vi "HWhist-TimeSeriesStrictTiming.vi"() -> ()   [LabVIEW 2017]
doc: "This example demonstrates how to use the Becker&Hickl LabVIEW wrapper VIs to acquire decay curves in continuous flow mode using the sequencer and swapping banks.\nMultiple modules are covered in a parallelized for loop.\nEach bank's decay curves are saved to a SDT-file on disc.\nThe SPC parameters can be adjusted for every new run. The rates and status flags are continuously updated. This VI is based on the C-example part 1 in use_spcm.c\n\ninfo@becker-hickl.com"
uses:
  Example_Controls/UserInput-PerModules.ctl
  Example_Controls/UserInput-AllModules.ctl
  SPC_Wrappers/SPC_Controls/ADCResolution.ctl
  SPC_Wrappers/SPC_Controls/StateCluster.ctl
  Example_Controls/CFM_States.ctl
  SPC_Wrappers/SPC_Controls/dither_range.ctl
  SPC_Wrappers/SPC_Controls/SPCdata.ctl
  SPC_Wrappers/SPC_Controls/macro_time_clk.ctl
  SPC_Wrappers/SPC_Controls/par_id.ctl
panel:
  out "Measurement Time":dbl(knob) scale=0.0..153.59999084472656
  out "CurrentBank":sgl
  out "SavingTime[s]":dbl
  out "saving":bool[](array[boolean])
  out "collecting":bool[](array[boolean])
  out "Busy":bool
  out "Sync Status":bool=TRUE
  in  "Tab Control":T1(tab)
  in  "User Input AllModules":T2={"tac_range"=50.033573, "tac_gain"=1, "tac_offset"=0.0, "tac_limit_high"=100.0, "tac_limit_low"=0.0, "collect_time"=0.1} {"tac_limit_high" min=0 max=100 step=0.1; "collect_time" min=1e-07 max=100000 step=0.001; "tac_offset" min=0 max=100 step=0.1; "tac_gain" min=1 max=15 step=1; "tac_range" format="%^#_6g"}
  in  "No of Routing Channels":i16(ring)=1 items=["1"=1, "2"=2, "3"=3, "4"=4, "5"=5, "6"=6, "7"=7, "8"=8, "9"=9, "10"=10, "11"=11, "12"=12, "13"=13, "14"=14, "15"=15, "16"=16]
  in  "ADC Resolution":T3=12 items=["1"=0, "4"=2, "16"=4, "64"=6, "256"=8, "1024"=10, "4096"=12]
  in  "User Input PerModule":T4[](array[typedef])=[{"sync_threshold"=-50.0, "sync_zc_level"=-5.2999988, "sync_freq_div"=1, "cfd_limit_low"=-50.0, "cfd_zc_level"=5.3000016}, {"sync_threshold"=-50.0, "sync_zc_level"=-5.2999988, "sync_freq_div"=1, "cfd_limit_low"=-50.0, "cfd_zc_level"=5.3}] {"sync_freq_div" items=["1"=1, "2"=2, "4"=4]; "cfd_zc_level" min=-96 max=96 step=0.1 format="%#_3g"; "cfd_limit_low" min=-500 max=0 step=0.1 format="%#_3g"; "sync_zc_level" min=-96 max=96 step=0.1 format="%#_3g"; "sync_threshold" min=-500 max=-20 step=0.1 format="%#_3g"}
  in  "Use First Entry\nFor All Modules":bool=TRUE
  out "Sync Array":T5(array[cluster])=[{"Sync Rate"=49999104.0, TRUE, "CFD Rate"=548976.0, "TAC Rate"=517664.0, "ADC Rate"=0.0}, {"Sync Rate"=49999360.0, TRUE, "CFD Rate"=544768.0, "TAC Rate"=514432.0, "ADC Rate"=0.0}]
  out "State Array":T6[](array[typedef])
  in  "ActiveModules":i32[](listbox)
  out "Data":u16[][](graph) caption="FirstCurve only"
  out "IntensityGraph":cluster{"Intensity Graph":u16[][]}[](array[cluster])
  in  "Saving Path":path=path "c:/temp"
  in  "Stop Application":bool
  out "Cycle Process":dbl(slide)=10.0 scale=0.0..100.0
  in  "CountCycles":bool=TRUE
  out "Current Cycle":i32=1
  in  "Number of\nCycles":i32=3
  in  "Stop Measurement":bool
  in  "Start Measurement":bool
  out "Started at":timestamp=timestamp(3689245583.9141345 s since 1904-01-01)
  out "Estimated Duration\nper Bank [min]":sgl=0.85333335
  out "Estimated Duration\nper Bank [s]":sgl=51.2
  out "Active Module No":i16[](array[numeric])=[0, 1]
  # "This example demonstrates how to use the Becker&Hickl LabVIEW wrapper VIs to acquire decay curves in continuous flow mode using the sequencer and swapping banks.\nMultiple modules are covered in a parallelized for loop.\nEach bank's decay curves are saved to a SDT-file on disc.\nThe SPC parameters can be adjusted for every new run. The rates and status flags are continuously updated.              This VI is based on the C-example part 1 in use_spcm.c."
  # "TAC / Time Range"
  # "range"
  # "gain"
  # "offset"
  # "limit high"
  # "limit low"
  # "Collection Time"
  # "CFD"
  # "(start)"
  # "SYNC"
  # "(stop)"
  # "threshold(LL)"
  # "zero cross(ZC)"
  # "See Tip-Strip for details"
  # "(c) 2022 Becker & Hickl GmbH\n     ALL RIGHTS RESERVED."
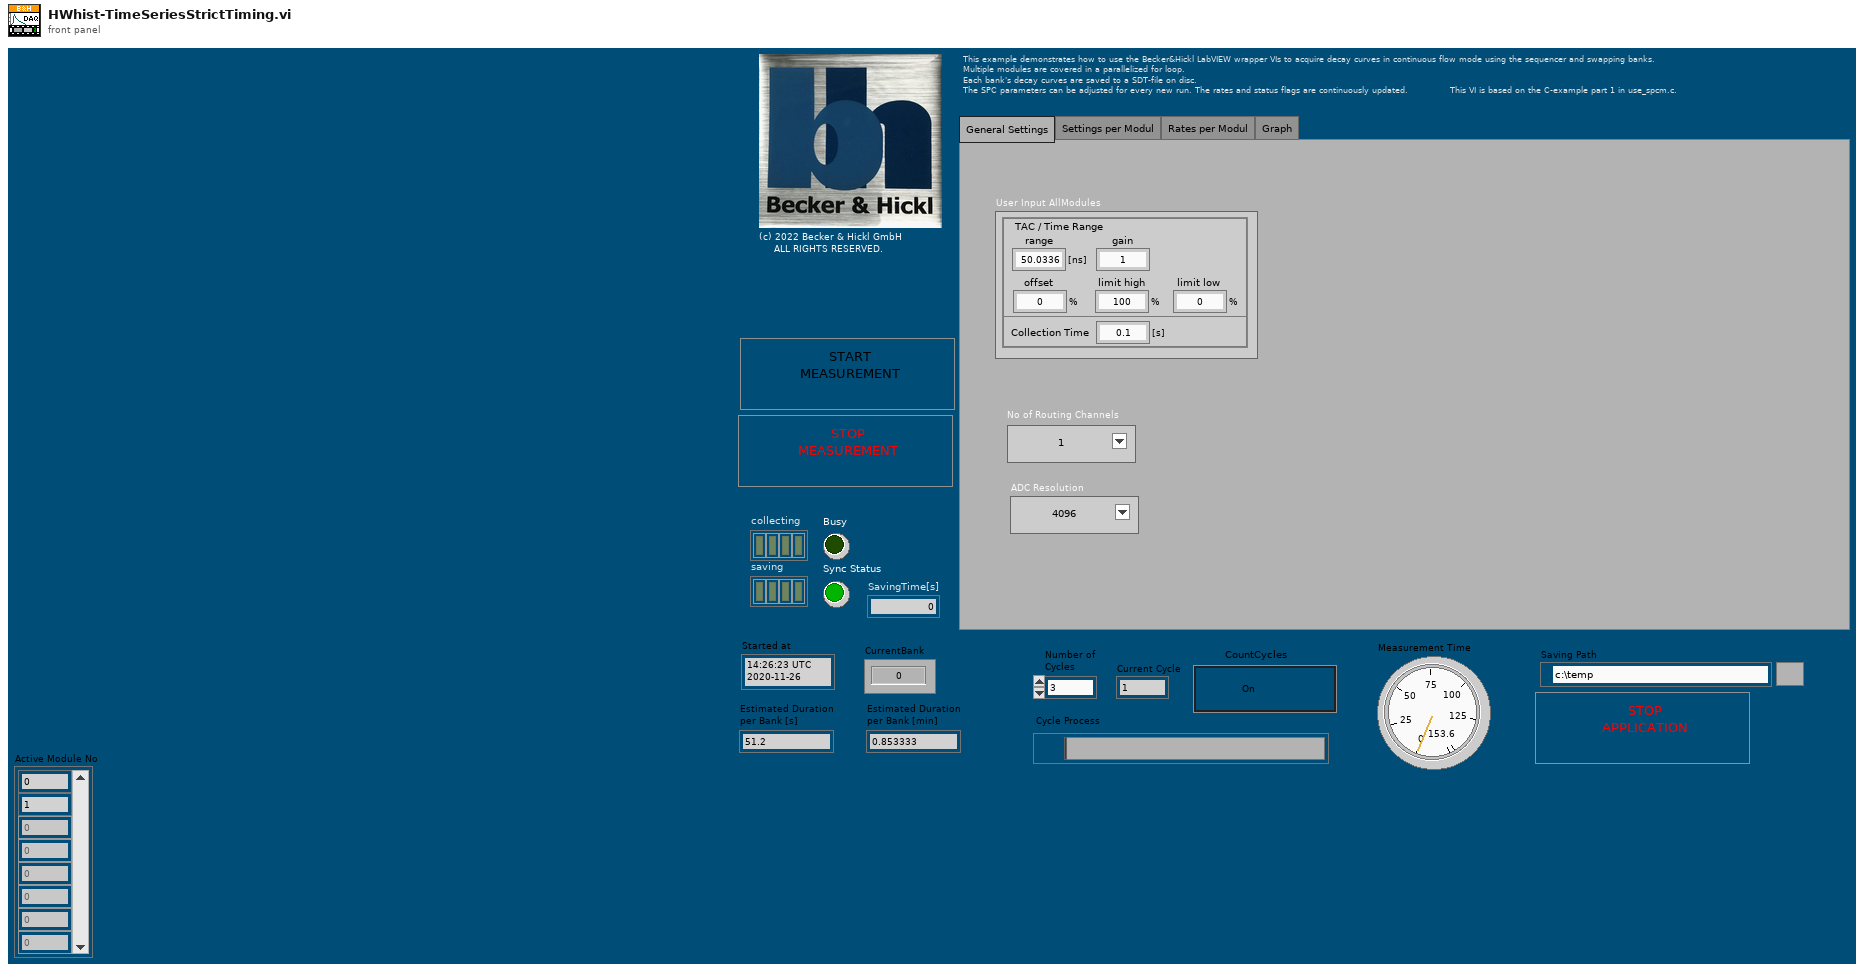
[diagram p1: front panel]
types:
  T1 = enum32{"General Settings", "Settings per Modul", "Rates per Modul", "Graph"}
  T2 = typedef "UserInput-AllModules.ctl" = cluster{"tac_range":sgl, "tac_gain":i16, "tac_offset":sgl, "tac_limit_high":sgl, "tac_limit_low":sgl, "collect_time":sgl}
  T3 = typedef "ADCResolution.ctl" = i16
  T4 = typedef "UserInput-PerModules.ctl" = cluster{"sync_threshold":sgl, "sync_zc_level":sgl, "sync_freq_div":i16, "cfd_limit_low":sgl, "cfd_zc_level":sgl}
  T5 = cluster{"Sync Rate":sgl, bool, "CFD Rate":sgl, "TAC Rate":sgl, "ADC Rate":sgl}[]
  T6 = typedef "StateCluster.ctl" = cluster{"OVERFL":bool, "OVERFLOW":bool, "TIME_OVER":bool, "COLTIM_OVER":bool, "CMD_STOP":bool, "ARMED":bool, "REPTIM_OVER":bool, "COLTIM_2OVER":bool, "REPTIM_2OVER":bool, "FOVFL":bool, "FEMPTY":bool, "FBRDY":bool, "SCRDY":bool, "MEASURE":bool, "WAIT_TRG":bool, "HFILL_NRDY":bool, "SEQ_STOP":bool, "SEQ_GAP150":bool, "WAIT_FR":bool}
  T7 = typedef "macro_time_clk.ctl" = enum16{"25ns", "Sync", "1/2 Sync", "1/4 Sync", "1/8 Sync"}
  T8 = typedef "SPCdata.ctl" = cluster{"base_adr":u16, "init":i16, "cfd_limit_low":sgl, "cfd_limit_high":sgl, "cfd_zc_level":sgl, "cfd_holdoff":sgl, "sync_zc_level":sgl, "sync_holdoff":sgl, "sync_threshold":sgl, "tac_range":sgl, "sync_freq_div":i16, "tac_gain":i16, "tac_offset":sgl, "tac_limit_low":sgl, "tac_limit_high":sgl, "adc_resolution":i16, "ext_latch_delay":i16, "collect_time":sgl, "display_time":sgl, "repeat_time":sgl, "stop_on_time":i16, "stop_on_ovfl":i16, "dither_range":i16, "count_incr":i16, "mem_bank":i16, "dead_time_comp":i16, "scan_control":u16, "routing_mode":u16, "tac_enable_hold":sgl, "pci_card_no":i16, "mode":u16, "scan_size_x":u32, "scan_size_y":u32, "scan_rout_x":u32, "scan_rout_y":u32, "scan_flyback":u32, "scan_borders":u32, "scan_polarity":u16, "pixel_clock":u16, "line_compression":u16, "trigger":u16, "pixel_time":sgl, "ext_pixclk_div":u32, "rate_count_time":sgl, "macro_time_clk":i16, "add_select":i16, "test_eep":i16, "adc_zoom":i16, "img_size_x":u32, "img_size_y":u32, "img_rout_x":u32, "img_rout_y":u32, "xy_gain":i16, "master_clock":i16, "adc_sample_delay":i16, "detector_type":i16, "chan_enable":u32, "chan_slope":u32, "chan_spec_no":u32, "tdc_control":u32, "tdc_offset1":sgl, "tdc_offset2":sgl, "tdc_offset3":sgl, "tdc_offset4":sgl, "tdc_offset5":sgl, "tdc_offset6":sgl, "cfd_th5_tdc":sgl, "cfd_th6_tdc":sgl, "cfd_zc5_tdc":sgl, "cfd_zc6_tdc":sgl, "future_reserve1":u64, "future_reserve2":u64, "future_reserve3":u64, "future_reserve4":u64}
  T9 = typedef "dither_range.ctl" = i16
  T10 = typedef "CFM_States.ctl" = enum16{"Init", "IDLE", "PrepareMeasurement", "StartMeasurement"}
  T11 = typedef "SPCModInfo.ctl" = cluster{"Module Type":T12, "Bus Number":i16, "Slot Number":i16, "in Use":i16, "Init Status":i16, "Base I/O Addr":u16}
  T12 = typedef "ModuleType.ctl" = i16
  T13 = typedef "ConfigMem.ctl" = cluster{"Max Block No":i32, "Blocks Per Frame":i32, "Frames Per Page":i32, "Maxpage":i32, "Block Length":i32}
  T14 = typedef "par_id.ctl" = i16
  T15 = typedef "SPC_RatesCluster.ctl" = cluster{"Sync":sgl, "CFD":sgl, "TAC":sgl, "ADC":sgl}
  T16 = cluster{"Sync":sgl, bool, "CFD":sgl, "TAC":sgl, "ADC":sgl}
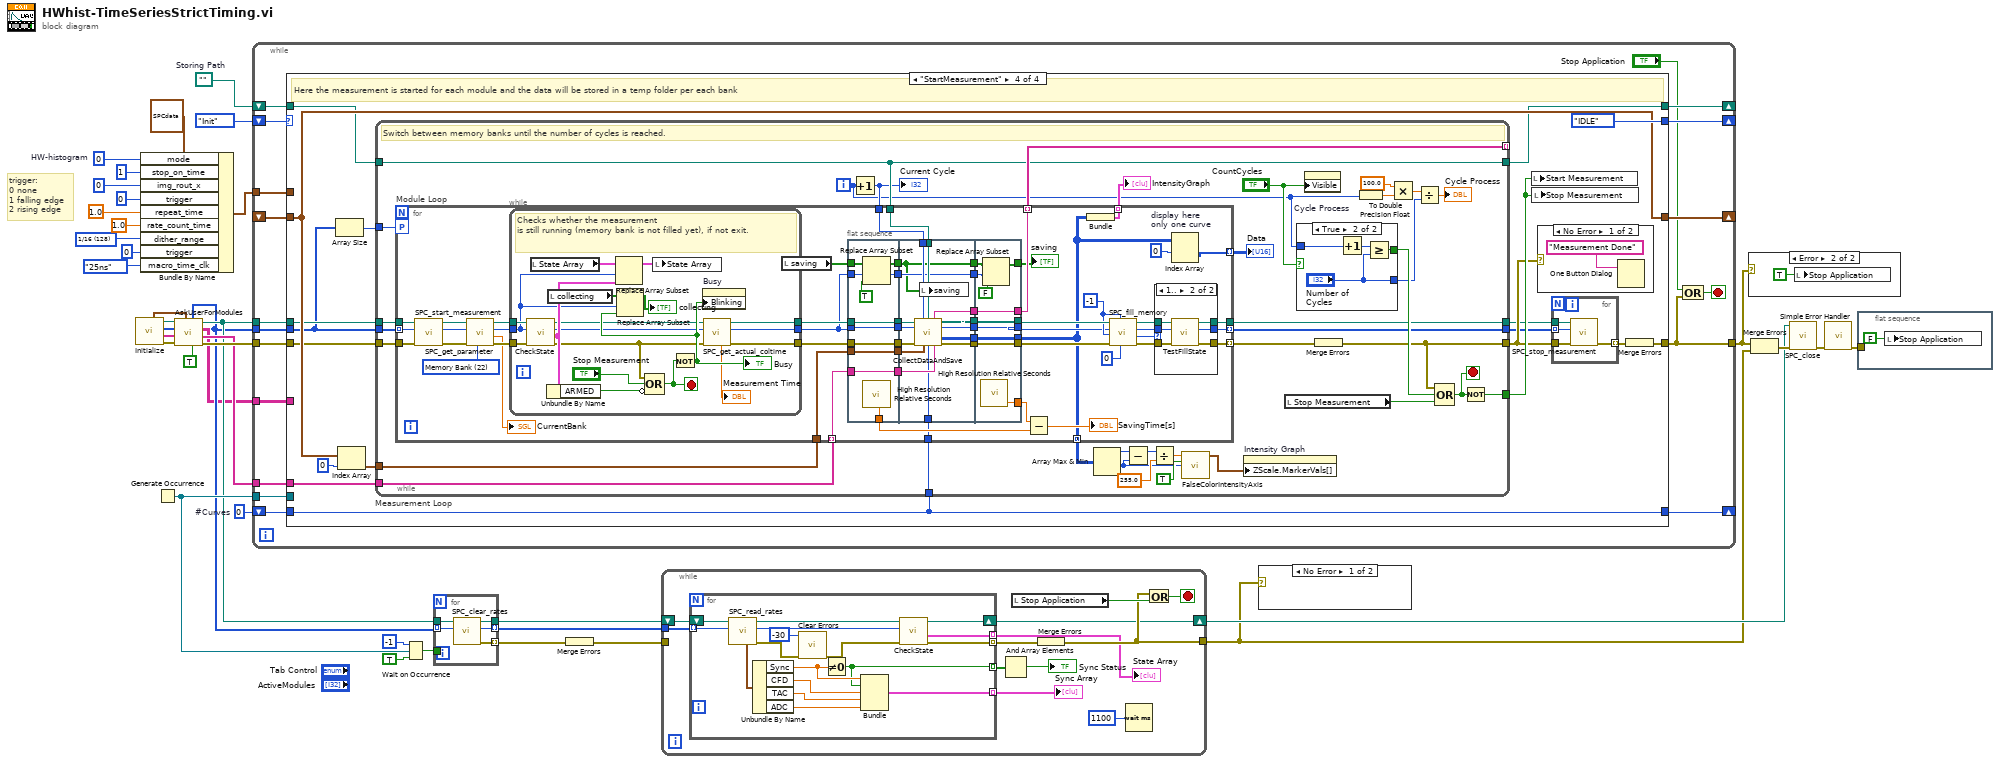
[diagram p0: block diagram]
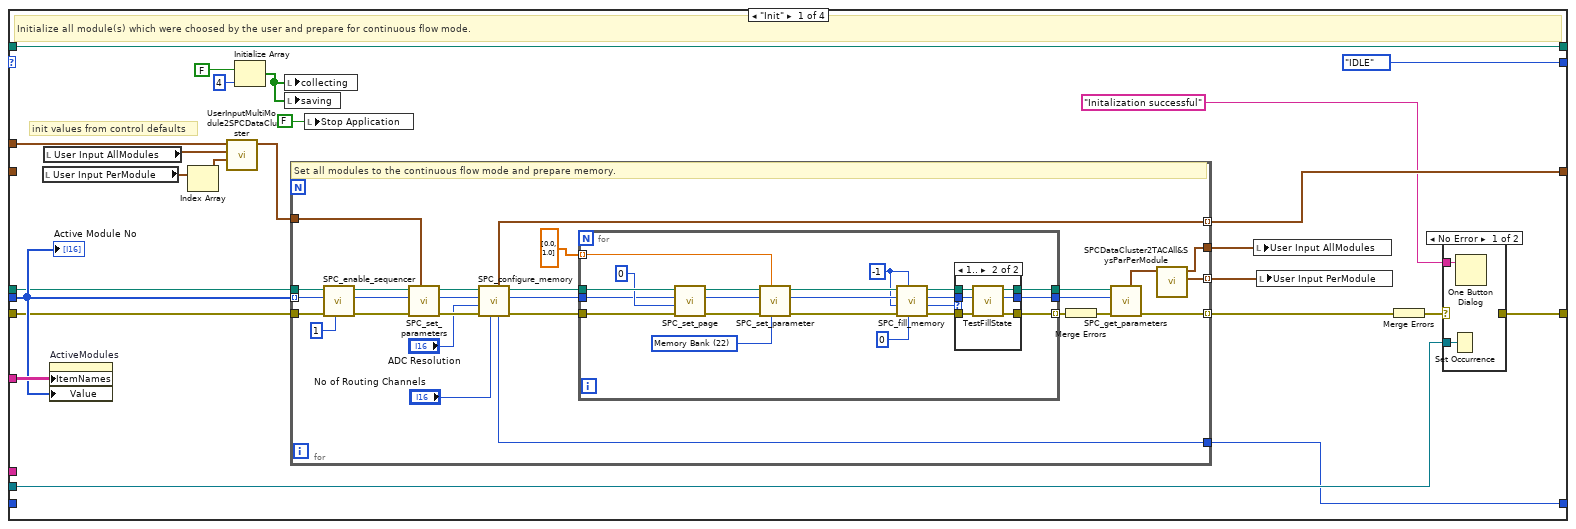
[diagram p2: hidden frame]
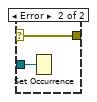
[diagram p3: hidden frame]
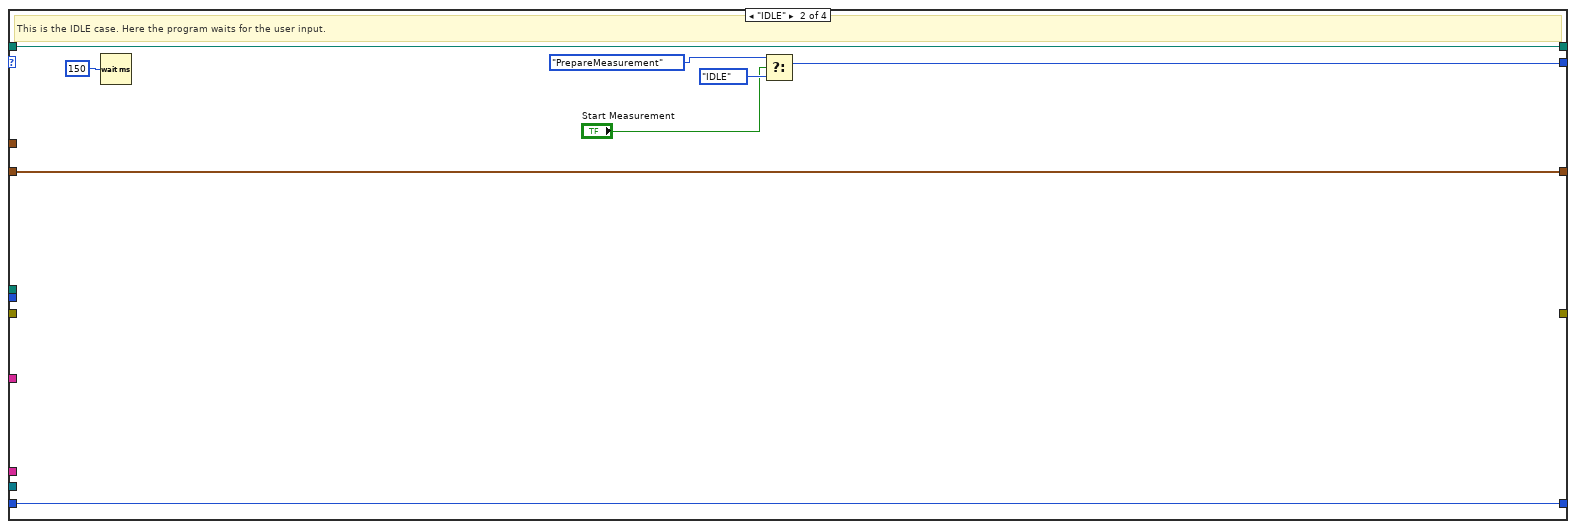
[diagram p5: hidden frame]
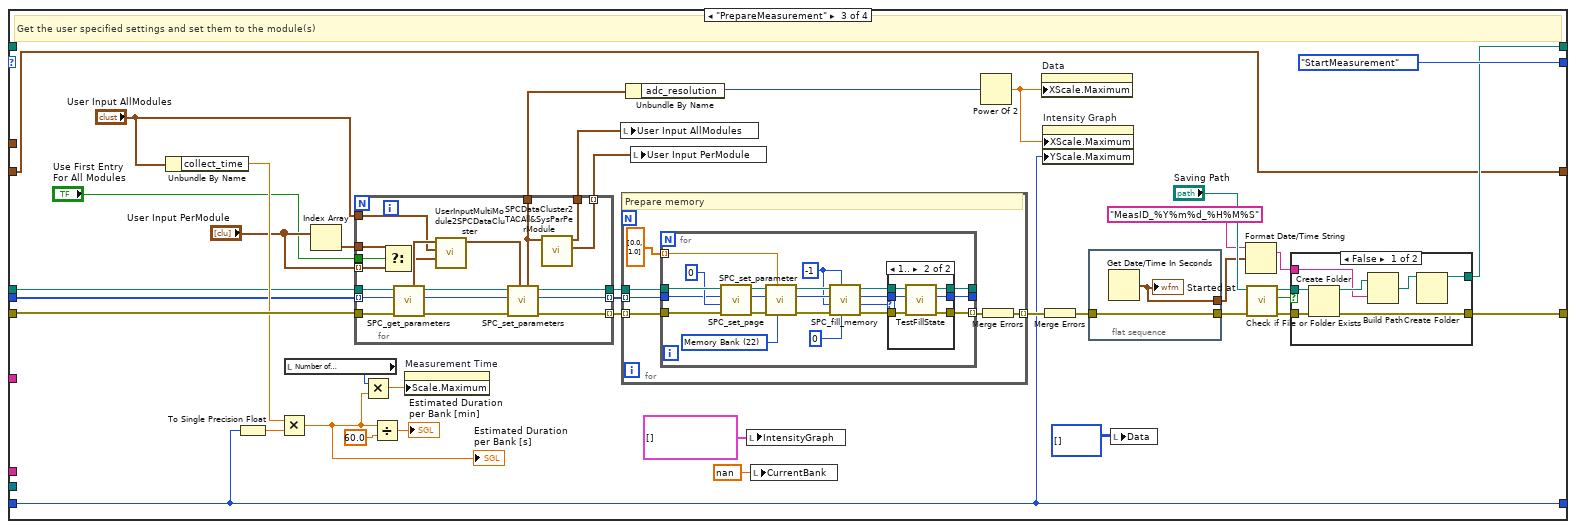
[diagram p6: hidden frame]
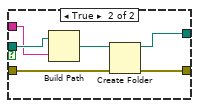
[diagram p8: hidden frame]
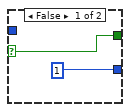
[diagram p11: hidden frame]
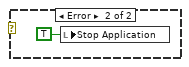
[diagram p12: hidden frame]
diagram:
  w4 = T9 128 items=["0"=0, "1/64"=32, "1/32"=64, "1/16"=128, "1/8"=256] ("DithRange")
  w12 = u16 0  # HW-histogram
  w17 = 0  # #Curves
  w35 = path ""  # Storing Path
  # "trigger:\n0 none\n1 falling edge\n2 rising edge"
  n1 = call "Initialize.vi"() -> ("ErrorOut"=w29:errorcluster, "SerialNumbersArray"=w24:string[], "ModuleNoArray"=w25:i16[], "DLL Path"=w33:path, "SPCModulesArray"=w23:T11[])  [unwired: 7 in]
  n2 = Bundle By Name(cluster=T8 {"base_adr"=896, "init"=0, "cfd_limit_low"=5.0, "cfd_limit_high"=80.0, "cfd_zc_level"=0.0, "cfd_holdoff"=5.0, "sync_zc_level"=0.0, "sync_holdoff"=4.0, "sync_threshold"=-20.0, "tac_range"=50.0, "sync_freq_div"=1, "tac_gain"=1, "tac_offset"=0.0, "tac_limit_low"=10.0, "tac_limit_high"=80.0, "adc_resolution"=10, "ext_latch_delay"=0, "collect_time"=0.01, "display_time"=1.0, "repeat_time"=10.0001, "stop_on_time"=1, "stop_on_ovfl"=1, "dither_range"=0, "count_incr"=1, "mem_bank"=0, "dead_time_comp"=1, "scan_control"=61440, "routing_mode"=0, "tac_enable_hold"=10.0, "pci_card_no"=-1, "mode"=0, "scan_size_x"=1, "scan_size_y"=1, "scan_rout_x"=1, "scan_rout_y"=1, "scan_flyback"=0, "scan_borders"=0, "scan_polarity"=0, "pixel_clock"=0, "line_compression"=1, "trigger"=0, "pixel_time"=5e-08, "ext_pixclk_div"=1, "rate_count_time"=1.0, "macro_time_clk"=0, "add_select"=0, "test_eep"=0, "adc_zoom"=0, "img_size_x"=1, "img_size_y"=1, "img_rout_x"=1, "img_rout_y"=1, "xy_gain"=1, "master_clock"=0, "adc_sample_delay"=0, "detector_type"=1, "chan_enable"=4191231, "chan_slope"=0, "chan_spec_no"=34835, "tdc_control"=0, "tdc_offset1"=0.0, "tdc_offset2"=0.0, "tdc_offset3"=0.0, "tdc_offset4"=0.0, "tdc_offset5"=0.0, "tdc_offset6"=0.0, "cfd_th5_tdc"=0.0, "cfd_th6_tdc"=0.0, "cfd_zc5_tdc"=0.0, "cfd_zc6_tdc"=0.0, "future_reserve1"=0, "future_reserve2"=0, "future_reserve3"=0, "future_reserve4"=0} ("SPCdata In"), "mode"=w12, "stop_on_time"=i16 1 ("Stop on Time"), "img_rout_x"=u32 0 ("Image Routing Size X"), "trigger"=u16 0 ("External Trigger Condition"), "repeat_time"=sgl 1.0 ("Repeat Time [s]"), "rate_count_time"=sgl 1.0 ("Repeat Time [s]"), "dither_range"=w4, "trigger"=u16 0, "macro_time_clk"=macro_time_clk."25ns") -> (w13:T8)
  n3 = Generate Occurrence() -> (w36:refnum<k4>)
  n4 = call "AskUserForModules.vi"("MultiModule"=TRUE ("SkipDialog"), "SPCModulesArray"=w23, "Error In"=w29, "Serial Number"=w24, "ModuleNoArray"=w25, "DLL Path"=w33) -> ("Error Out"=w32:errorcluster, "ActiveSerialNumbers"=w22:string[], "ModuleListboxStrings"=w6:string[][], "DLL Path"=w19:path, "ActiveModuleNo"=w18:i16[])  [unwired: 1 in]
  n5 = while {
    shift-right: [w56] -> _
    shift-left: CFM_States."Init" ("CFM States") -> [w57]
    tunnel: w36 -> [w51]
    shift-right: [w50] -> _
    shift-left: _ -> [w49]
    shift-right: [w48] -> _
    shift-left: w17 -> [w47]
    shift-right: [w46] -> _
    shift-left: w35 -> [w45]
    tunnel: w18 -> [w43]
    tunnel: w22 -> [w42]
    tunnel: w32 -> [w54]
    tunnel: [w52] -> w15
    tunnel: w19 -> [w55]
    tunnel: w13 -> [w41]
    tunnel: w6 -> [w40]
    stop <- w53 stop-if-true
    n6 = case shown="\"StartMeasurement\"" w57 {
      tunnel: [CFM_States."IDLE" ("CFM States") w150 CFM_States."StartMeasurement" ("CFM States") CFM_States."IDLE" ("CFM States")] -> w56
      tunnel: [w75 _ w178 w262] -> w52
      tunnel: w55 -> [w59 _ w176 w269]
      tunnel: w54 -> [w58 _ w186 w267]
      tunnel: w51 -> [w80 _ _ _]
      tunnel: [w79 w146 w175 w277] -> w50
      tunnel: w49 -> [_ w146 w175 w277]
      tunnel: [w77 w145 w154 w261] -> w48
      tunnel: w47 -> [_ w145 w154 w261]
      tunnel: [w78 w144 w179 w275] -> w46
      tunnel: w45 -> [w78 w144 _ w276]
      tunnel: w43 -> [w61 _ w184 w268]
      tunnel: w42 -> [_ _ _ w272]
      tunnel: w41 -> [w64 _ _ _]
      tunnel: w40 -> [w62 _ _ _]
      frame "Init" {
        # "init values from control defaults"
        # "Initialize all module(s) which were choosed by the user and prepare for continuous flow mode."
        n7 = local read "User Input PerModule"() -> (w66:T4[])
        n8 = local read "User Input AllModules"() -> (w65:T2)
        n9 = property on="ActiveModules" class="MCListbox (strict)"("ItemNames"=w62, "Value"=w61) -> ()  [unwired: 2 in, 2 out]
        n10 = Index Array(array=w66) -> (element=w67:T4)  [unwired: 1 in]
        n11 = call "UserInputMultiModule2SPCDataCluster.vi"("User Input PerModules"=w67, "User Input AllModules"=w65, "SPCData_In"=w64) -> ("SPCData_Out"=w63:T8)  [unwired: 8 in]
        n12 = Initialize Array(FALSE, 4 ("dimension size")) -> (w74:bool[])
        n13 = local write "collecting"(w74) -> ()
        n14 = local write "saving"(w74) -> ()
        n15 = for {
          tunnel: w59 -> [w91]
          tunnel: w61 -> [w89] mode=indexing
          tunnel: w58 -> [w87]
          tunnel: [w104] -> w70 mode=indexing
          tunnel: w63 -> [w108]
          tunnel: [w106] -> w79 mode=indexing
          tunnel: [w93] -> w77
          tunnel: [w95] -> w69
          tunnel: [w94] -> w68 mode=indexing
          # "Set all modules to the continuous flow mode and prepare memory."
          n16 = call "SPC_enable_sequencer.vi"("Enable"=i16 1, "Error In"=w87, "Module No"=w89, "DLL Path"=w91) -> ("Error Out"=w86:errorcluster, "Module No"=w88:i16, "DLL Path"=w90:path)  [unwired: 5 in]
          n17 = call "SPC_set_parameters.vi"("SPCdata In"=w108, "Error In"=w86, "Module No."=w88, "DLL Path"=w90) -> ("Error Out"=w109:errorcluster, "Module No"=w110:i16, "DLL Path"=w111:path)  [unwired: 4 in, 1 out]
          n18 = call "SPC_configure_memory.vi"("No of Routing\nChannels"="No of Routing Channels", "Error In"=w109, "ADC Resolution [exponent]"="ADC Resolution", "Module No"=w110, "DLL Path"=w111) -> ("Error Out"=w100:errorcluster, "Module No"=w98:i16, "DLL Path"=w99:path, "#CurvesPerBank"=w93:i32, "SPCMemConfig"=w106:T13)  [unwired: 2 in]
          n19 = for {
            tunnel: sgl[] [0.0, 1.0] ("Parameter Value") -> [w133] mode=indexing
            tunnel: w100 -> [w124]
            tunnel: w98 -> [w121]
            tunnel: w99 -> [w123]
            tunnel: [w131] -> w103
            tunnel: [w114] -> w107 mode=indexing
            tunnel: [w132] -> w102
            w113 = T14 22 items=["CFD Limit Low", "CFD Limit High", "CFD Zero Cross Level", "CFD Holdoff", "SYNC Zero Cross Level", "SYNC Freq Divider", "SYNC Holdoff", "SYNC Threshold", "TAC Range", "TAC Gain", "TAC Offset", "TAC Limit Low", "TAC Limit High", "ADC Resolution", "External Latch Delay", "Collect Time", "Display Time", "Repeat Time", "Stop On Time", "Stop On Overflow", "Dither Range", "Count Increment", "Memory Bank", "Dead Time Compensation", "Scan Control", "Routing Mode", "TAC Enable Hold", "Operation Mode", "Scan Size X", "Scan Size Y", "Scan Routing X Bits", "Scan Routing Y Bits", "Scan Polarity", "Scan Flyback", "Scan Borders", "Pixel Time", "Pixel Clock Source", "Scan Line Compression", "External Trigger Condition", "External Pixel Clock Divider", "Rate Counting Time", "Macro Time Clock", "ADD Signal Source", "ADC Zoom", "XY Gain", "Image Size X", "Image Size Y", "Image Routing X Bits", "Image Routing Y Bits", "Master Clock", "ADC Sample Delay", "Detector Type", "X Axis Type", "Channel Enable", "Channel Slope", "Channel Spec_no"] ("SPC parameter ID")
            w115 = -1 ("Block to be filled")
            n20 = call "SPC_set_page.vi"("Error In"=w124, "Page"=0, "Module No"=w121, "DLL Path"=w123) -> ("Error Out"=w127:errorcluster, "Module No"=w126:i16, "DLL Path"=w125:path)  [unwired: 4 in, 1 out]
            n21 = call "SPC_set_parameter.vi"("SPC parameter ID"=w113, "Parameter Value"=w133, "Error In"=w127, "Module no"=w126, "DLL Path"=w125) -> ("Error Out"=w128:errorcluster, "Module no"=w129:i16, "DLL Path"=w130:path)  [unwired: 3 in, 1 out]
            n22 = call "SPC_fill_memory.vi"("Fill Value"=u16 0 ("Fill value"), "Block to be Filled"=w115, "Error In"=w128, "Page"=w115, "Module No"=w129, "DLL Path"=w130) -> ("Error Out"=w118:errorcluster, "FunctionReturn"=w116:i16, "Module No"=w119:i16, "DLL Path"=w120:path)  [unwired: 2 in]
            n23 = case shown="1.." w116 {
              tunnel: w120 -> [w136 w142]
              tunnel: w119 -> [w135 w141]
              tunnel: w118 -> [w134 w140]
              tunnel: [w136 w139] -> w131
              tunnel: [w134 w138] -> w114
              tunnel: [w135 w137] -> w132
              frame 0, Default {
              }
              frame 1.. {
                n24 = call "TestFillState.vi"("Error In"=w140, "Module No"=w141, "DLL Path"=w142) -> ("Error Out"=w138:errorcluster, "Module No"=w137:i16, "DLL Path"=w139:path)  [unwired: 6 in]
              }
            }
          }
          n25 = Merge Errors(w107) -> (w105:errorcluster)
          n26 = call "SPC_get_parameters.vi"("Error In"=w105, "Module No"=w102, "DLL Path"=w103) -> ("Error Out"=w104:errorcluster, "SPCdata"=w96:T8)  [unwired: 5 in, 2 out]
          n27 = call "SPCDataCluster2TACAll&SysParPerModule.vi"("SPCdata In"=w96) -> ("User Input PerModules"=w94:T4, "User Input AllModules"=w95:T2)  [unwired: 9 in]
        }
        n28 = local write "Stop Application"(FALSE) -> ()
        n29 = local write "User Input AllModules"(w69) -> ()
        n30 = local write "User Input PerModule"(w68) -> ()
        n31 = Merge Errors(w70) -> (w71:errorcluster)
        n32 = case shown="No Error" w71 {
          selector: w71 -> [_ w84]
          tunnel: w80 -> [w83 w85]
          tunnel: "Initalization successful" -> [w82 _]
          tunnel: [_ w84] -> w75
          frame No Error {
            n33 = Set Occurrence(w83) -> ()
            n34 = One Button Dialog(message=w82) -> ()  [unwired: 1 in, 1 out]
          }
          frame Error {
            n35 = Set Occurrence(w85) -> ()
          }
        }
        "Active Module No" <- w61
      }
      frame "IDLE" {
        # "This is the IDLE case. Here the program waits for the user input."
        n36 = Wait (ms)(milliseconds to wait=u32 150) -> ()  [unwired: 1 out]
        n37 = Select(t=CFM_States."PrepareMeasurement" ("CFM States"), s="Start Measurement", f=CFM_States."IDLE" ("CFM States")) -> (s? t:f=w150:T10)
      }
      frame "PrepareMeasurement" {
        # "Get the user specified settings and set them to the module(s)"
        n38 = Unbundle By Name("User Input AllModules") -> ("collect_time"=w185:sgl)
        n39 = To Single Precision Float(number=w154) -> (single precision float=w187:sgl)
        n40 = Multiply(x=w185, y=w187) -> (x*y=w157:sgl)
        "Estimated Duration\nper Bank [s]" <- w157
        n41 = local read "Number of\nCycles"() -> (w158:i32)
        n42 = Index Array(array="User Input PerModule") -> (element=w165:T4)  [unwired: 1 in]
        n43 = for {
          tunnel: w184 -> [w258] mode=indexing
          tunnel: w186 -> [w259]
          tunnel: w176 -> [w260]
          tunnel: [w254] -> w163
          tunnel: [w253] -> w169 mode=indexing
          tunnel: "User Input AllModules" -> [w251]
          tunnel: "User Input PerModule" -> [w249] mode=indexing
          tunnel: "Use First Entry\nFor All Modules" -> [w248]
          tunnel: w165 -> [w247]
          tunnel: [w245] -> w162
          tunnel: [w244] -> w153
          tunnel: [w243] -> w152 mode=indexing
          tunnel: [w242] -> w151 mode=indexing
          n44 = Select(t=w247, s=w248, f=w249) -> (s? t:f=w250:T4)
          n45 = call "SPC_get_parameters.vi"("Error In"=w259, "Module No"=w258, "DLL Path"=w260) -> ("Error Out"=w255:errorcluster, "Module No"=w256:i16, "DLL Path"=w257:path, "SPCdata"=w252:T8)  [unwired: 5 in]
          n46 = call "UserInputMultiModule2SPCDataCluster.vi"("User Input PerModules"=w250, "User Input AllModules"=w251, "SPCData_In"=w252) -> ("SPCData_Out"=w246:T8)  [unwired: 8 in]
          n47 = call "SPC_set_parameters.vi"("SPCdata In"=w246, "Error In"=w255, "Module No."=w256, "DLL Path"=w257) -> ("Error Out"=w242:errorcluster, "Module No"=w243:i16, "DLL Path"=w244:path, "SPCdata Out"=w245:T8)  [unwired: 4 in]
          n48 = call "SPCDataCluster2TACAll&SysParPerModule.vi"("SPCdata In"=w245) -> ("User Input PerModules"=w253:T4, "User Input AllModules"=w254:T2)  [unwired: 9 in]
        }
        n49 = Multiply(x=w158, y=w157) -> (x*y=w159:sgl)
        n50 = Divide(x=w157, y=sgl 60.0) -> (x/y=→"Estimated Duration\nper Bank [min]":sgl)
        n51 = property on="Measurement Time" class="Knob (strict)"("Scale.Maximum"=w159) -> ()  [unwired: 2 in, 2 out]
        n52 = local write "User Input AllModules"(w163) -> ()
        n53 = for {
          tunnel: [w194] -> w156 mode=indexing
          tunnel: w153 -> [w193]
          tunnel: w152 -> [w192] mode=indexing
          tunnel: w151 -> [w191] mode=indexing
          # "Prepare memory"
          n54 = for {
            tunnel: sgl[] [0.0, 1.0] ("Parameter Value") -> [w217] mode=indexing
            tunnel: w191 -> [w208]
            tunnel: w192 -> [w205]
            tunnel: w193 -> [w207]
            tunnel: [w215] -> _
            tunnel: [w198] -> w195 mode=indexing
            tunnel: [w216] -> _
            w197 = T14 22 items=["CFD Limit Low", "CFD Limit High", "CFD Zero Cross Level", "CFD Holdoff", "SYNC Zero Cross Level", "SYNC Freq Divider", "SYNC Holdoff", "SYNC Threshold", "TAC Range", "TAC Gain", "TAC Offset", "TAC Limit Low", "TAC Limit High", "ADC Resolution", "External Latch Delay", "Collect Time", "Display Time", "Repeat Time", "Stop On Time", "Stop On Overflow", "Dither Range", "Count Increment", "Memory Bank", "Dead Time Compensation", "Scan Control", "Routing Mode", "TAC Enable Hold", "Operation Mode", "Scan Size X", "Scan Size Y", "Scan Routing X Bits", "Scan Routing Y Bits", "Scan Polarity", "Scan Flyback", "Scan Borders", "Pixel Time", "Pixel Clock Source", "Scan Line Compression", "External Trigger Condition", "External Pixel Clock Divider", "Rate Counting Time", "Macro Time Clock", "ADD Signal Source", "ADC Zoom", "XY Gain", "Image Size X", "Image Size Y", "Image Routing X Bits", "Image Routing Y Bits", "Master Clock", "ADC Sample Delay", "Detector Type", "X Axis Type", "Channel Enable", "Channel Slope", "Channel Spec_no"] ("SPC parameter ID")
            w199 = -1 ("Block to be filled")
            n55 = call "SPC_set_page.vi"("Error In"=w208, "Page"=0, "Module No"=w205, "DLL Path"=w207) -> ("Error Out"=w211:errorcluster, "Module No"=w210:i16, "DLL Path"=w209:path)  [unwired: 4 in, 1 out]
            n56 = call "SPC_set_parameter.vi"("SPC parameter ID"=w197, "Parameter Value"=w217, "Error In"=w211, "Module no"=w210, "DLL Path"=w209) -> ("Error Out"=w212:errorcluster, "Module no"=w213:i16, "DLL Path"=w214:path)  [unwired: 3 in, 1 out]
            n57 = call "SPC_fill_memory.vi"("Fill Value"=u16 0 ("Fill value"), "Block to be Filled"=w199, "Error In"=w212, "Page"=w199, "Module No"=w213, "DLL Path"=w214) -> ("Error Out"=w202:errorcluster, "FunctionReturn"=w200:i16, "Module No"=w203:i16, "DLL Path"=w204:path)  [unwired: 2 in]
            n58 = case shown="1.." w200 {
              tunnel: w204 -> [w220 w226]
              tunnel: w203 -> [w219 w225]
              tunnel: w202 -> [w218 w224]
              tunnel: [w220 w223] -> w215
              tunnel: [w218 w222] -> w198
              tunnel: [w219 w221] -> w216
              frame 0, Default {
              }
              frame 1.. {
                n59 = call "TestFillState.vi"("Error In"=w224, "Module No"=w225, "DLL Path"=w226) -> ("Error Out"=w222:errorcluster, "Module No"=w221:i16, "DLL Path"=w223:path)  [unwired: 6 in]
              }
            }
          }
          n60 = Merge Errors(w195) -> (w194:errorcluster)
        }
        n61 = Unbundle By Name(w162) -> ("adc_resolution"=w161:i16)
        n62 = local write "User Input PerModule"(w169) -> ()
        n63 = local write "IntensityGraph"(cluster{"Intensity Graph":u16[][]}[] [] ("IntensityGraph")) -> ()
        n64 = local write "CurrentBank"(sgl nan ("CurrentBank")) -> ()
        n65 = Power Of 2(x=w161) -> (2^x=w160:dbl)
        n66 = property on="Data" class="WFGraph (strict)"("XScale.Maximum"=w160) -> ()  [unwired: 2 in, 2 out]
        n67 = property on="Intensity Graph" class="IntGraph (strict)"("XScale.Maximum"=w160, "YScale.Maximum"=w154) -> ()  [unwired: 2 in, 2 out]
        n68 = Merge Errors(w156) -> (w155:errorcluster)
        n69 = flat-sequence {
          tunnel: w155 -> [w240]
          tunnel: [w241] -> w173
          tunnel: [w240] -> w177
          frame #0 {
            n70 = Get Date/Time In Seconds() -> (seconds since 1Jan1904=w241:timestamp)
            "Started at" <- w241
          }
        }
        n71 = local write "Data"(u16[][] [] ("Data")) -> ()
        n72 = Format Date/Time String(time format string (%c)="MeasID_%Y%m%d_%H%M%S", seconds (now)=w173) -> (date/time string=w172:string)  [unwired: 1 in]
        n73 = call <vilib>:"Check if File or Folder Exists.vi"("error in (no error)"=w177, "path"="Saving Path") -> ("error out"=w180:errorcluster, "file or folder exists?"=w182:bool, "dup path"=w181:path)  [unwired: 7 in]
        n74 = case shown="False" w182 {
          tunnel: w181 -> [w233 w239]
          tunnel: w180 -> [w232 w237]
          tunnel: [w231 w236] -> w178
          tunnel: [w228 w235] -> w179
          tunnel: w172 -> [w227 w234]
          frame False {
            n75 = Create Folder(path (use dialog)=w233, error in=w232) -> (created path=w229:path, error out=w231:errorcluster)  [unwired: 1 in, 1 out]
            n76 = Build Path(base path=w229, name or relative path=w227) -> (appended path=w230:path)
            n77 = Create Folder(path (use dialog)=w230) -> (created path=w228:path)  [unwired: 2 in, 2 out]
          }
          frame True {
            n78 = Build Path(base path=w239, name or relative path=w234) -> (appended path=w238:path)
            n79 = Create Folder(path (use dialog)=w238, error in=w237) -> (created path=w235:path, error out=w236:errorcluster)  [unwired: 1 in, 1 out]
          }
        }
      }
      frame "StartMeasurement" {
        # "Here the measurement is started for each module and the data will be stored in a temp folder per each bank"
        n80 = Array Size(array=w268) -> (size(s)=w270:i32)
        n81 = Index Array(array=w277, index=0) -> (element=w274:T13)
        n82 = while "Measurement Loop" {
          tunnel: [w301] -> w265
          tunnel: w268 -> [w304]
          tunnel: w274 -> [w303]
          tunnel: w261 -> [w284]
          tunnel: w276 -> [w302]
          tunnel: [w302] -> w275
          tunnel: [w315] -> _ mode=indexing
          tunnel: w270 -> [w285]
          tunnel: [w313] -> w271
          tunnel: w272 -> [w312]
          tunnel: w267 -> [w306]
          tunnel: w269 -> [w305]
          tunnel: [w300] -> w264
          tunnel: [w299] -> w263
          i -> [w286]
          stop <- w314 stop-if-true
          # "Switch between memory banks until the number of cycles is reached."
          n83 = Increment(x=w286) -> (x+1=w298:i32)
          "Current Cycle" <- w298
          n84 = for "Module Loop" {
            tunnel: [w329] -> w317 mode=indexing
            tunnel: [w372] -> w315 mode=indexing
            tunnel: w312 -> [w371] mode=indexing
            tunnel: w306 -> [w331]
            tunnel: w305 -> [w334]
            tunnel: w304 -> [w326] mode=indexing
            tunnel: w303 -> [w366]
            tunnel: w302 -> [w365]
            tunnel: [w328] -> w300
            tunnel: [w327] -> w299 mode=indexing
            tunnel: w298 -> [w324]
            tunnel: [w323] -> w297 mode=indexing
            tunnel: [w321] -> w295 mode=indexing
            tunnel: [w320] -> w287 mode=concatenating
            workers-P: w285 -> [_]
            tunnel: w284 -> [w319]
            w358 = -1 ("Block to be Filled")
            w369 = T14 22 items=["CFD Limit Low", "CFD Limit High", "CFD Zero Cross Level", "CFD Holdoff", "SYNC Zero Cross Level", "SYNC Freq Divider", "SYNC Holdoff", "SYNC Threshold", "TAC Range", "TAC Gain", "TAC Offset", "TAC Limit Low", "TAC Limit High", "ADC Resolution", "External Latch Delay", "Collect Time", "Display Time", "Repeat Time", "Stop On Time", "Stop On Overflow", "Dither Range", "Count Increment", "Memory Bank", "Dead Time Compensation", "Scan Control", "Routing Mode", "TAC Enable Hold", "Operation Mode", "Scan Size X", "Scan Size Y", "Scan Routing X Bits", "Scan Routing Y Bits", "Scan Polarity", "Scan Flyback", "Scan Borders", "Pixel Time", "Pixel Clock Source", "Scan Line Compression", "External Trigger Condition", "External Pixel Clock Divider", "Rate Counting Time", "Macro Time Clock", "ADD Signal Source", "ADC Zoom", "XY Gain", "Image Size X", "Image Size Y", "Image Routing X Bits", "Image Routing Y Bits", "Master Clock", "ADC Sample Delay", "Detector Type", "X Axis Type", "Channel Enable", "Channel Slope", "Channel Spec_no"] ("SPC parameter ID")
            n85 = call "SPC_start_measurement.vi"("Error In"=w331, "Module No"=w326, "DLL Path"=w334) -> ("Error Out"=w330:errorcluster, "Module No"=w332:i16, "DLL Path"=w333:path)  [unwired: 6 in]
            n86 = call "SPC_get_parameter.vi"("SPC Parameter ID"=w369, "Error In"=w330, "Module No"=w332, "DLL Path"=w333) -> ("Error Out"=w368:errorcluster, "Current Parameter Value"=→"CurrentBank":sgl, "Module No"=w349:i16, "DLL Path"=w367:path)  [unwired: 4 in]
            n87 = while {
              tunnel: [w421] -> w335
              tunnel: [w419] -> w336
              tunnel: w368 -> [w430]
              tunnel: w349 -> [w425]
              tunnel: w367 -> [w431]
              tunnel: [w420] -> w322
              stop <- w436 stop-if-true
              # "Checks whether the measurement\nis still running (memory bank is not filled yet), if not exit."
              n88 = call "CheckState.vi"("Error In"=w430, "Module No."=w425, "DLL Path"=w431) -> ("Error Out"=w422:errorcluster, "SPC_StateCluster"=w428:T6, "Module No."=w423:i16, "DLL Path"=w424:path)  [unwired: 4 in, 1 out]
              n89 = local read "State Array"() -> (w427:T6[])
              n90 = Unbundle By Name(w428) -> ("ARMED"=w429:bool)
              n91 = local read "collecting"() -> (w434:bool[])
              n92 = Replace Array Subset(array=w427, new element=w428, index=w425) -> (w426:T6[])
              n93 = Compound Arithmetic op=OR(w422, "Stop Measurement", invert w429) -> (w436:bool)
              n94 = local write "State Array"(w426) -> ()
              n95 = Not(x=w436) -> (.not. x?=w432:bool)
              "Busy" <- w432
              n96 = Replace Array Subset(array=w434, new element=w432, index=w425) -> (→"collecting":bool[])
              n97 = property on="Busy" class="Bool (strict)"("Blinking"=w432) -> ()  [unwired: 2 in, 2 out]
              n98 = call "SPC_get_actual_coltime.vi"("Error In"=w422, "Module No"=w423, "DLL Path"=w424) -> ("Error Out"=w419:errorcluster, "Module No"=w420:i16, "DLL Path"=w421:path, "coltime"=→"Measurement Time":sgl)  [unwired: 5 in]
            }
            n99 = local read "saving"() -> (w357:bool[])
            n100 = flat-sequence {
              tunnel: w322 -> [w375]
              tunnel: w357 -> [w377]
              tunnel: w336 -> [w379]
              tunnel: w366 -> [w380]
              tunnel: w322 -> [w381]
              tunnel: w371 -> [w382]
              tunnel: w335 -> [w383]
              tunnel: [w383] -> w346
              tunnel: [w382] -> w345
              tunnel: [w381] -> w344
              tunnel: [w380] -> w343
              tunnel: [w379] -> w342
              tunnel: [w375] -> w341
              tunnel: [w378] -> w339
              tunnel: [w376] -> w337
              tunnel: w365 -> [w390]
              tunnel: w324 -> [w389]
              tunnel: [w397] -> w356
              tunnel: [w396] -> w355
              tunnel: [w394] -> w354
              tunnel: [w393] -> w353
              tunnel: [w385] -> w352
              tunnel: [w387] -> w351
              tunnel: [w386] -> w348
              tunnel: w346 -> [w398]
              tunnel: w345 -> [w395]
              tunnel: w344 -> [w392]
              tunnel: w343 -> [w391]
              tunnel: w342 -> [w388]
              tunnel: w341 -> [w387]
              tunnel: w337 -> [w385]
              tunnel: w319 -> [w384]
              tunnel: [w401] -> w350
              tunnel: [w405] -> w320
              tunnel: [w406] -> w370
              tunnel: [w407] -> w372
              tunnel: [w408] -> w373
              tunnel: w356 -> [w408]
              tunnel: w355 -> [w407]
              tunnel: w354 -> [w406]
              tunnel: w353 -> [w405]
              tunnel: w352 -> [w404]
              tunnel: w351 -> [w403]
              tunnel: [w400] -> w347
              tunnel: w348 -> [w400]
              tunnel: [w399] -> w340
              frame #0 {
                n101 = Replace Array Subset(array=w377, new element=TRUE ("new element/subarray"), index=w375) -> (w376:bool[])
                n102 = call <vilib>:"High Resolution Relative Seconds.vi"() -> ("relative seconds"=w378:dbl)
              }
              frame #1 {
                n103 = call "CollectDataAndSave.vi"("SPC DLL Path"=w398, "CycleNo"=w389, "Storing Path"=w390, "Module No"=w392, "error in"=w388, "SPC memory config"=w391, "#Curves"=w384, "Serialnumber\nper Module"=w395) -> ("stored to"=w396:string, "SPC DLL Path"=w397:path, "Module No"=w386:i16, "Data"=w393:u16[][], "error out"=w394:errorcluster)  [unwired: 3 in]
                n104 = local write "saving"(w385) -> ()
              }
              frame #2 {
                n105 = call <vilib>:"High Resolution Relative Seconds.vi"() -> ("relative seconds"=w399:dbl)
                n106 = Replace Array Subset(array=w404, new element=FALSE ("new element/subarray"), index=w403) -> (w401:bool[])
              }
            }
            n107 = Subtract(x=w340, y=w339) -> (x-y=→"SavingTime[s]":dbl)
            n108 = Bundle("Data"=w320) -> (w323:cluster{"Data":u16[][]})  [unwired: 1 in]
            n109 = call "SPC_fill_memory.vi"("Fill Value"=u16 0 ("Fill value"), "Block to be Filled"=w358, "Error In"=w370, "Page"=w358, "Module No"=w347, "DLL Path"=w373) -> ("Error Out"=w361:errorcluster, "FunctionReturn"=w359:i16, "Module No"=w362:i16, "DLL Path"=w363:path)  [unwired: 2 in]
            n110 = case shown="1.." w359 {
              tunnel: w363 -> [w410 w417]
              tunnel: w362 -> [w409 w416]
              tunnel: w361 -> [w411 w415]
              tunnel: [w411 w414] -> w329
              tunnel: [w410 w413] -> w328
              tunnel: [w409 w412] -> w327
              frame 0, Default {
              }
              frame 1.. {
                n111 = call "TestFillState.vi"("Error In"=w415, "Module No"=w416, "DLL Path"=w417) -> ("Error Out"=w414:errorcluster, "Module No"=w412:i16, "DLL Path"=w413:path)  [unwired: 6 in]
              }
            }
            n112 = Index Array "display here\nonly one curve"(array=w320, index (row)=0) -> (element=w321:u16[])  [unwired: 1 in]
            "saving" <- w350
          }
          "IntensityGraph" <- w297
          "Data" <- w295
          n113 = Array Max & Min(array=w287) -> (max value=w292:u16, min value=w288:u16)  [unwired: 2 out]
          n114 = Subtract(x=w292, y=w288) -> (x-y=w289:u16)
          n115 = Divide(x=w289, y=255.0) -> (x/y=w291:dbl)
          n116 = call "FalseColorIntensityAxis.vi"("Offset"=w288, "ViewColor"=TRUE, "Scale"=w291) -> ("ZScaleMarkerVals"=w294:cluster{dbl, "Color Box":u32}[])  [unwired: 8 in]
          n117 = property on="Intensity Graph" class="IntGraph (strict)"("ZScale.MarkerVals[]"=w294) -> ()  [unwired: 2 in, 2 out]
          n118 = local read "Stop Measurement"() -> (w316:bool)
          n119 = case shown="True" "CountCycles" {
            selector: "CountCycles" -> [w438 _]
            tunnel: [w438 w442] -> w318
            tunnel: w286 -> [_ w441]
            tunnel: [1 "Number of\nCycles"] -> w309
            frame False {
            }
            frame True {
              n120 = Increment(x=w441) -> (x+1=w439:i32)
              n121 = Greater Or Equal?(x=w439, y="Number of\nCycles") -> (x >= y?=w442:bool)
            }
          }
          n122 = property on="Cycle Process" class="Slide (strict)"("Visible"="CountCycles") -> ()  [unwired: 2 in, 2 out]
          n123 = Merge Errors(w317) -> (w301:errorcluster)
          n124 = To Double Precision Float(number=w286) -> (double precision float=w307:dbl)
          n125 = Multiply(x=100.0, y=w307) -> (x*y=w310:dbl)
          n126 = Divide(x=w310, y=w309) -> (x/y=→"Cycle Process":dbl)
          n127 = Compound Arithmetic op=OR(w301, w318, w316) -> (w314:bool)
          n128 = Not(x=w314) -> (.not. x?=w313:bool)
        }
        n129 = local write "Start Measurement"(w271) -> ()
        n130 = local write "Stop Measurement"(w271) -> ()
        n131 = case shown="No Error" w265 {
          frame No Error {
            n132 = One Button Dialog(message="Measurement Done") -> ()  [unwired: 1 in, 1 out]
          }
          frame Error {
          }
        }
        n133 = for {
          tunnel: w264 -> [w280]
          tunnel: w263 -> [w279] mode=indexing
          tunnel: w265 -> [w281]
          tunnel: [w282] -> w266 mode=indexing
          n134 = call "SPC_stop_measurement.vi"("Error In"=w281, "Module No"=w279, "DLL Path"=w280) -> ("Error Out"=w282:errorcluster)  [unwired: 6 in, 2 out]
        }
        n135 = Merge Errors(w266) -> (w262:errorcluster)
      }
    }
    n136 = Compound Arithmetic op=OR("Stop Application", w52) -> (w53:bool)
  }
  n137 = Wait on Occurrence(1:TRUE, 2:w36, 3:-1) -> (0:w21:bool)
  n138 = for {
    tunnel: w19 -> [w447]
    tunnel: [w446] -> w27
    tunnel: w18 -> [w445] mode=indexing
    tunnel: [w444] -> w28 mode=indexing
    tunnel: [w443] -> w34 mode=indexing
    tunnel: w21 -> [_]
    n139 = call "SPC_clear_rates.vi"("Module no"=w445, "DLL Path"=w447) -> ("Error Out"=w444:errorcluster, "Module  No"=w443:i16, "DLL Path"=w446:path)  [unwired: 7 in]
  }
  n140 = Merge Errors(w28) -> (w26:errorcluster)
  n141 = while {
    tunnel: w34 -> [w458]
    tunnel: w26 -> [_]
    tunnel: [w451] -> w16
    shift-right: [w450] -> w20
    shift-left: w27 -> [w459]
    stop <- w453 stop-if-true
    n142 = for {
      tunnel: w458 -> [w466] mode=indexing
      tunnel: [w469] -> w455 mode=indexing
      tunnel: [w470] -> w454 mode=indexing
      shift-right: [w464] -> w450
      shift-left: w459 -> [w476]
      tunnel: [w461] -> w449 mode=indexing
      tunnel: [w460] -> w448 mode=indexing
      n143 = call "SPC_read_rates.vi"("Module No"=w466, "DLL Path"=w476) -> ("Error Out"=w467:errorcluster, "Module No"=w463:i16, "DLL Path"=w465:path, "SPC_RatesCluster"=w475:T15)  [unwired: 6 in]
      n144 = Unbundle By Name(w475) -> ("Sync"=w474:sgl, "CFD"=w473:sgl, "TAC"=w472:sgl, "ADC"=w471:sgl)
      n145 = call <vilib>:"Clear Errors.vi"("error in (no error)"=w467, "specific error code to clear (0: all)"=-30) -> ("error out"=w462:errorcluster)  [unwired: 4 in, 1 out]
      n146 = Not Equal To 0?(x=w474) -> (x != 0?=w469:bool)
      n147 = Bundle("Sync"=w474, w469, "CFD"=w473, "TAC"=w472, "ADC"=w471) -> (w470:T16)  [unwired: 1 in]
      n148 = call "CheckState.vi"("Error In"=w462, "Module No."=w463, "DLL Path"=w465) -> ("Error Out"=w461:errorcluster, "SPC_StateCluster"=w460:T6, "DLL Path"=w464:path)  [unwired: 4 in, 2 out]
    }
    "Sync Array" <- w454
    "State Array" <- w448
    n149 = And Array Elements(Boolean array=w455) -> (logical AND=→"Sync Status":bool)
    n150 = local read "Stop Application"() -> (w452:bool)
    n151 = Merge Errors(w449) -> (w451:errorcluster)
    n152 = Wait (ms)(milliseconds to wait=u32 1100) -> ()  [unwired: 1 out]
    n153 = Or(x=w451, y=w452) -> (x .or. y?=w453:bool)
  }
  n154 = case shown="No Error" w16 {
    frame No Error {
    }
    frame Error {
      n155 = local write "Stop Application"(TRUE ("Stop Application")) -> ()
    }
  }
  n156 = case shown="Error" w15 {
    frame No Error {
    }
    frame Error {
      n157 = local write "Stop Application"(TRUE ("Stop Application")) -> ()
    }
  }
  n158 = Merge Errors(w15, w16) -> (w30:errorcluster)
  n159 = call "SPC_close.vi"("Error In"=w30, "DLL Path"=w20) -> ("Error Out"=w31:errorcluster)  [unwired: 8 in, 1 out]
  n160 = call <vilib>:"Simple Error Handler.vi"("error in (no error)"=w31) -> ("error out"=w14:errorcluster)  [unwired: 4 in, 4 out]
  n161 = flat-sequence {
    tunnel: w14 -> [_]
    frame #0 {
      n162 = local write "Stop Application"(FALSE ("Stop Application")) -> ()
    }
  }
